vi "comm config.vi"(4 "Stop Bits":u16(ring)=10 items=["1.0"=10, "1.5"=15, "2.0"=20], 6 "Parity":u16(ring) items=["None", "Odd", "Even", "Mark", "Space"], 8 "error in (no error)":errorcluster, 9 "Data Bits":u16=8, 10 "Baud Rate":u32=9600, 11 "Comm Handle":u64) -> (0 "error out":errorcluster, 3 "dup Comm Handle":u64)   [LabVIEW 2024, in "lvserial.lvlib"]
doc: "Sets the basic comunication parameters (baud rate, data bits, parity and stop bits) for a specified communications device."
uses:
  <instrlib>/lvserial/lvserial.lvlib
  lvserial.dll
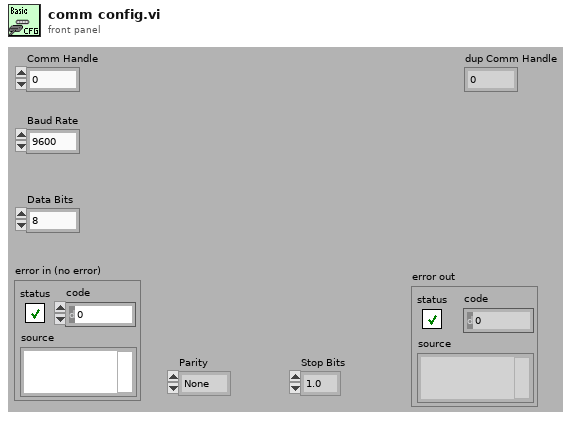
[diagram p1: front panel]
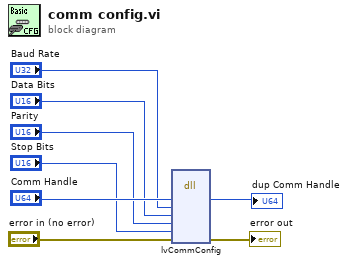
[diagram p0: block diagram]
diagram:
  n1 = dll-call lib="lvserial.dll" fn="lvCommConfig"("hComm"="Comm Handle", "ulBaudRate"="Baud Rate", "usDataBits"="Data Bits", "usParity"="Parity", "usStopBits"="Stop Bits", "error"="error in (no error)") -> ("hComm"=→"dup Comm Handle":u64, "error"=→"error out":errorcluster)  [unwired: 7 in, 3 out]
